vi "CEXT.vi"(1 "Numeric Input":cxt format="%.2f") -> (0 "Numeric Output":cxt format="%.2f")   [LabVIEW 2012]
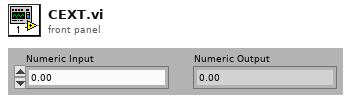
[diagram p1: front panel]
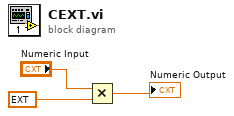
[diagram p0: block diagram]
diagram:
  n1 = Multiply(x="Numeric Input", y=ext 2.0) -> (x*y=→"Numeric Output":cxt)
